vi "max_regelung.vi"(5 "TI 21a IW °C":dbl, 9 "TI 21a SW °C":dbl=60.0 min=30.0 max=60.0, 10 "Öl-Regelung":bool, 11 "TI 02 IW °C":dbl) -> (2 "zu":bool=TRUE, 3 "auf":bool=TRUE)   [LabVIEW 2015]
panel:
  in  "OK":bool
  in  "Totzeit":dbl=6.0
  in  "PT1 Faktor":dbl=2.0000000000000004
  in  "PT1 Tau":dbl=10.0
  in  "SP2":dbl=-0.15
  in  "SP4":dbl=0.2
  in  "SP1":dbl=-0.2
  in  "SP3":dbl=0.15
  # "Regelparameter"
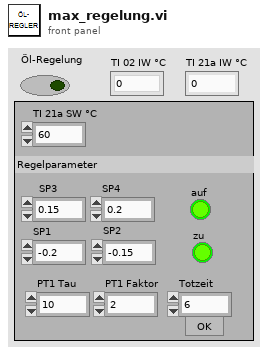
[diagram p1: front panel]
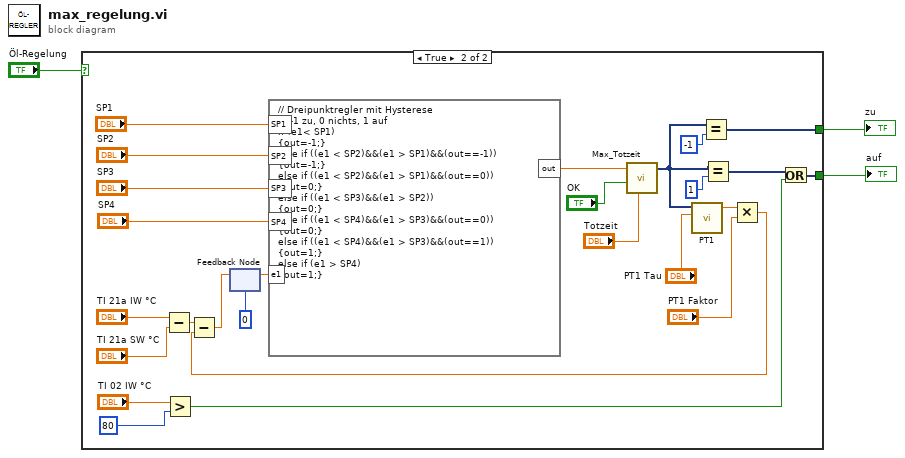
[diagram p0: block diagram]
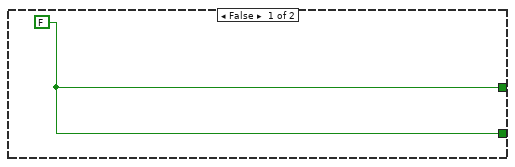
[diagram p2: hidden frame]
diagram:
  n1 = case shown="True" "Öl-Regelung" {
    tunnel: [w4 w26] -> w2
    tunnel: [w4 w12] -> w1
    frame False {
      w4 = FALSE
    }
    frame True {
      n2 = Subtract(x="TI 21a IW °C", y="TI 21a SW °C") -> (x-y=w20:dbl)
      n3 = Greater?(x="TI 02 IW °C", y=80) -> (0:w11:bool)
      n4 = feedback #1(0) -> (w17:dbl)
      n5 = formula code="// Dreipunktregler mit Hysterese\n//  -1 zu, 0 nichts, 1 auf\nif (e1< SP1)\n{out=-1;}\nelse if ((e1 < SP2)&&(e1 > SP1)&&(out==-1))\n{out=-1;}\nelse if ((e1 < SP2)&&(e1 > SP1)&&(out==0))\n{out=0;}\nelse if ((e1 < SP3)&&(e1 > SP2))\n{out=0;}\nelse if ((e1 < SP4)&&(e1 > SP3)&&(out==0))\n{out=0;}\nelse if ((e1 < SP4)&&(e1 > SP3)&&(out==1))\n{out=1;}\nelse if (e1 > SP4)\n{out=1;}"("e1"=w17, "SP1"="SP1", "SP3"="SP3", "SP4"="SP4", "SP2"="SP2") -> ("out"=w8:dbl)
      n6 = call "Max_Totzeit.vi"("Totzeit"="Totzeit", "Reset"="OK", "Signals"=w8) -> ("Delayed Signals"=w7:dynamicdata)  [unwired: 7 in, 1 out]
      n7 = call "PT1.vi"("Zeitkonstante(Tau)"="PT1 Tau", "Eingang"=w7) -> ("Ausgang"=w10:dbl)  [unwired: 9 in]
      n8 = Equal?(x=w7, y=-1) -> (x = y?=w26:dynamicdata)
      n9 = Equal?(x=w7, y=1) -> (x = y?=w13:dynamicdata)
      n10 = Multiply(x=w10, y="PT1 Faktor") -> (x*y=w19:dbl)
      n11 = Subtract(x=w20, y=w19) -> (x-y=w18:dbl)
      n12 = feedback-in #1(w18) -> ()
      n13 = Or(x=w13, y=w11) -> (x .or. y?=w12:dynamicdata)
    }
  }
  "zu" <- w2
  "auf" <- w1
